vi "2.3.-Lectura de Imagen - Operador Umbral.vi"() -> ()   [LabVIEW 2020]
panel:
  in  "Umbral R":u64(slide) scale=0.0..255.0
  in  "Umbral B":u64(slide) scale=0.0..255.0
  out "new picture":picture
  in  "Path":path
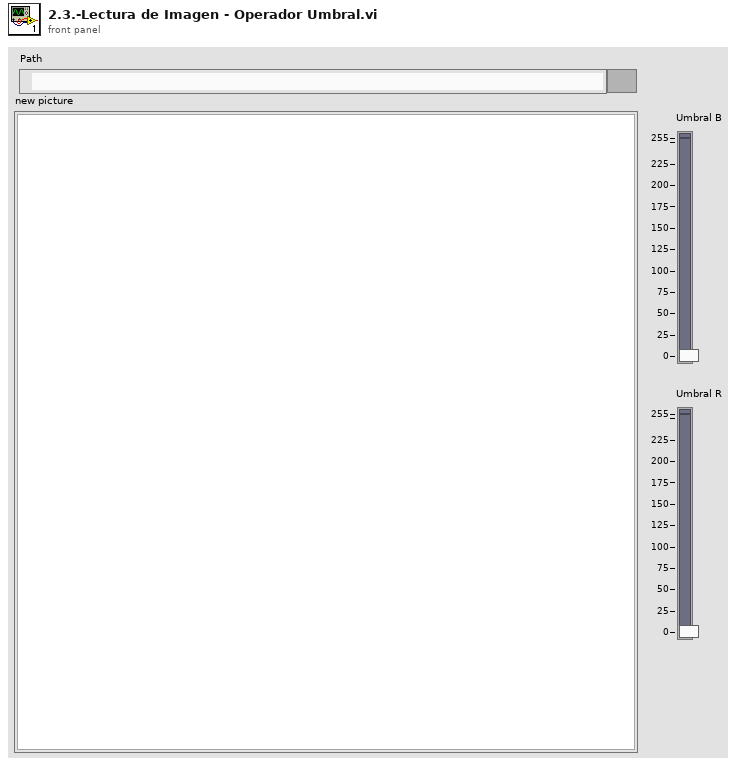
[diagram p1: front panel]
types:
  T1 = typedef "imagedata.ctl" = cluster{"image type":i32, "image depth":i32, "image":u8[], "mask":u8[], "colors":u32[], "Rectangle":cluster{"left":i16, "top":i16, "right":i16, "bottom":i16}}
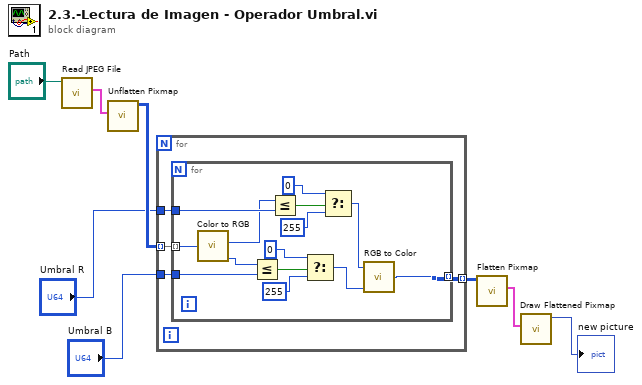
[diagram p0: block diagram]
diagram:
  n1 = call <vilib>:"Read JPEG File.vi"("path to JPEG file"="Path") -> ("image data"=w7:T1)  [unwired: 8 in, 2 out]
  n2 = call <vilib>:"Unflatten Pixmap.vi"("image data"=w7) -> ("24-bit pixmap"=w6:u32[][])  [unwired: 4 in, 6 out]
  n3 = for {
    tunnel: w6 -> [w12] mode=indexing
    tunnel: [w11] -> w5 mode=indexing
    tunnel: "Umbral B" -> [w10]
    tunnel: "Umbral R" -> [w9]
    n4 = for {
      tunnel: w12 -> [w26] mode=indexing
      tunnel: [w25] -> w11 mode=indexing
      tunnel: w10 -> [w22]
      tunnel: w9 -> [w17]
      n5 = call <vilib>:"Color to RGB.vi"("Color"=w26) -> ("R"=w13:u8, "B"=w14:u8)  [unwired: 2 out]
      n6 = Less Or Equal?(x=w14, y=w22) -> (x <= y?=w21:bool)
      n7 = Less Or Equal?(x=w13, y=w17) -> (x <= y?=w20:bool)
      n8 = Select(t=0, s=w21, f=255) -> (s? t:f=w15:i32)
      n9 = Select(t=0, s=w20, f=255) -> (s? t:f=w16:i32)
      n10 = call <vilib>:"RGB to Color.vi"("B"=w15, "R"=w16) -> ("Color"=w25:u32)  [unwired: 1 in]
    }
  }
  n11 = call <vilib>:"Flatten Pixmap.vi"("24-bit pixmap"=w5) -> ("image data"=w4:T1)  [unwired: 10 in]
  n12 = call <vilib>:"Draw Flattened Pixmap.vi"("image data"=w4) -> ("new picture"=→"new picture":picture)  [unwired: 8 in]
